vi "Begin.vi"(8 "error in (no error)":errorcluster, 11 "DriverXBoxController in":refnum<class "DriverXBoxController.lvclass">) -> (0 "error out":errorcluster, 3 "DriverXBoxController out":refnum<class "DriverXBoxController.lvclass">)   [LabVIEW 2013, in "DriverXBoxController.lvclass"]
uses:
  DriverXBoxController.lvclass
  <vilib>/Rock Robotics/WPI/Joystick/WPI_JoystickDeviceEnum.ctl
  XboxController/XBoxController.lvclass
  XboxController/XBoxController.lvclass/XBoxController.ctl
  <vilib>/Rock Robotics/WPI/Joystick/WPI_JoystickOpen.vi
panel:
  in  "JoystickDevice":T1=enum."USB 2"
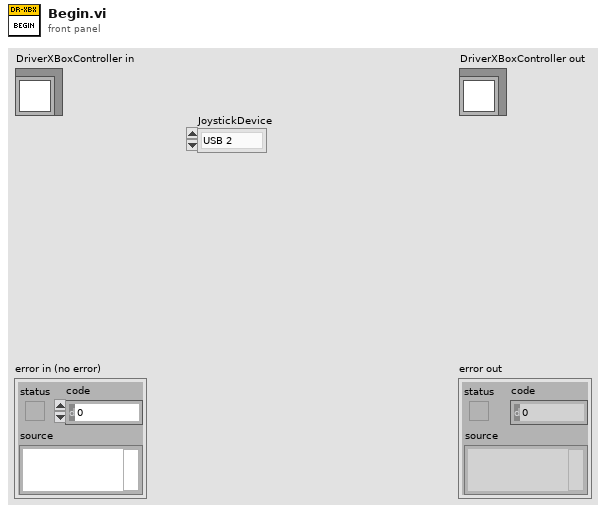
[diagram p1: front panel]
types:
  T1 = typedef "WPI_JoystickDeviceEnum.ctl" = enum16{"USB 1", "USB 2", "USB 3", "USB 4", "Kinect 1", "Kinect 2"}
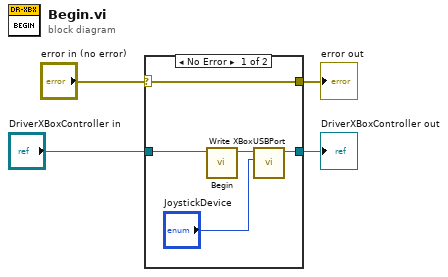
[diagram p0: block diagram]
diagram:
  n1 = case shown="No Error" "error in (no error)" {
    selector: "error in (no error)" -> [w9 w10]
    tunnel: [w9 w10] -> w3
    tunnel: "DriverXBoxController in" -> [w8 w11]
    tunnel: [w6 w11] -> w1
    frame No Error {
      n2 = call-parent "Begin.vi"("XBoxController in"=w8) -> ("XBoxController out"=w7:refnum<class "DriverXBoxController.lvclass">)  [unwired: 9 in, 1 out]
      n3 = call "Write XBoxUSBPort.vi"("XBoxUSBPort"="JoystickDevice", "XBoxController in"=w7) -> ("XBoxController out"=w6:refnum<class "DriverXBoxController.lvclass">)  [unwired: 8 in, 1 out]
    }
    frame Error {
    }
  }
  "error out" <- w3
  "DriverXBoxController out" <- w1
